vi "nanocal-frontend-server.vi"() -> ()   [LabVIEW 2020]
uses:
  icicle.ctl
  publisher action.ctl
  NanoCalLib 20210521/MCL.lvlibp/SynkTek FPGA/FPGA_SharedResources/FPGASharedResources_Readings_ReadingChannelTypedef.ctl
  NanoCalLib 20210521/MCL.lvlibp/SynkTek FPGA/FPGA_SharedResources/FPGASharedResources_Lockin_Typedef.ctl
  NanoCalLib 20210521/MCL.lvlibp/SynkTek FPGA/FPGA_SharedResources/FPGASharedResources_PhaseType_Typedef.ctl
  NanoCalLib 20210521/NanoCalLib.lvlibp
  NanoCalLib 20210521/MCL.lvlibp/SynkTek FPGA/FPGA_SharedResources/FPGA_SharedResources.lvlib
  NanoCalLib 20210521/MCL.lvlibp
panel:
  in  "Tab Control":enum32{"Page 1", "Page 2"}(tab)
  in  "wait (ms)":u32=50
  out "nanocal data":T1[](array[typedef])=[{"name"="frequency", "units"="Hz", "data"=22.999983439900642}, {"name"="Cs/T", "units"="J/K^2", "data"=3.7739249893269324e-24}, {"name"="Ts", "units"="K", "data"=0.01038672245174747}, {"name"="Ts^2", "units"="K^2", "data"=0.00010788400328963498}, {"name"="Tr", "units"="K", "data"=0.010160855980464388}, {"name"="Cs", "units"="J/K", "data"=3.9198711417852884e-26}, {"name"="Cr", "units"="J/K", "data"=-2.0417082109734875e-18}, {"name"="Ks", "units"="W/K", "data"=2.527872170547633e-23}, {"name"="Kr", "units"="W/K", "data"=3.911459306754245e-15}, {"name"="Rs-therm", "units"="Ohm", "data"=81348.62911437088}, {"name"="Rr-therm", "units"="Ohm", "data"=196009.13306498667}, {"name"="Cr/T", "units"="J/K^2", "data"=-2.0093860348960226e-16}, {"name"="dlogR/dlogT -- S ", "units"="a.u.", "data"=0.8738049990739949}, {"name"="tau", "units"="s", "data"=0.001550660348832471}, {"name"="tan(phi)", "units"="a.u", "data"=0.4481816480367121}, {"name"="Ts,ac", "units"="K", "data"=0.1660718459124116}, {"name"="Tr,ac", "units"="K", "data"=0.0}, {"name"="Hs,ac,out", "units"="V", "data"=0.0}, {"name"="Offset,dc,out", "units"="V", "data"=1.0000000009313226}, {"name"="Vdiff,ac", "units"="V", "data"=4.688238574611993e-09}, {"name"="Vdiff,ac,phase", "units"="deg", "data"=82.61397850464}, {"name"="Stherm,ac,out", "units"="V", "data"=0.0}, {"name"="Rtherm,ac,out", "units"="V", "data"=0.0}, {"name"="CV1 -- Re", "units"="V", "data"=6.026901987025408e-10}, {"name"="CV1 -- Im", "units"="V", "data"=4.649338174070346e-09}, {"name"="DV2 -- Re", "units"="V", "data"=1.0380460195223816e-09}, {"name"="DV2 -- Im", "units"="V", "data"=6.197949303499005e-09}, {"name"="AV2 -- Re", "units"="V", "data"=6.687727898351347e-10}, {"name"="AV2 -- Im", "units"="V", "data"=1.6238645509657183e-10}, {"name"="Vdiff,norm, Re", "units"="V", "data"=1.298136411917629e+18}, {"name"="Vdiff,norm, Im", "units"="V", "data"=1.00142248672243e+19}, {"name"="Resistance.RHr", "units"="ohm", "data"=501162.54690786166}, {"name"="Resistance.RHs", "units"="ohm", "data"=286805.4208747116}]
  in  "Stop":bool
  # "nanocal -- frontend server"
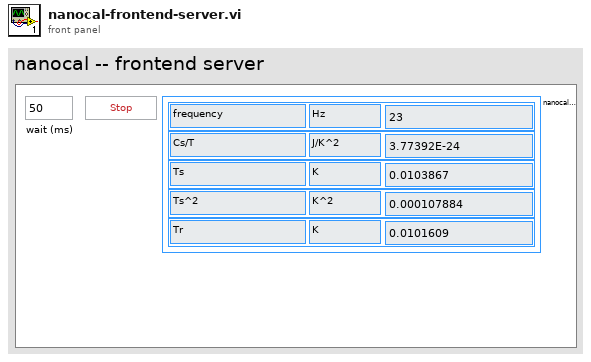
[diagram p1: front panel]
types:
  T1 = typedef "icicle.ctl" = cluster{"name":string, "units":string, "data":dbl}
  T2 = typedef "MCL.lvlibp/MCL_DataRef.ctl" = refnum<vi>
  T3 = typedef "MCL.lvlibp/FPGA_SharedResources.lvlib/FPGASharedResources_PhaseType_Typedef.ctl" = enum16{"DC", "X", "Y", "R", "Theta"}
  T4 = typedef "publisher action.ctl" = enum16{"set", "get", "init", "check"}
  T5 = typedef "MCL.lvlibp/FPGA_SharedResources.lvlib/FPGASharedResources_Lockin_Typedef.ctl" = enum8{"Lock-in set L1", "Lock-in set L2"}
  T6 = typedef "MCL.lvlibp/FPGA_SharedResources.lvlib/FPGASharedResources_Readings_ReadingChannelTypedef.ctl" = enum8{"A V1", "A V2", "B V1", "B V2", "C V1", "C V2", "D V1", "D V2", "E V1", "E V2", "A I", "B I", "C I", "D I", "E I", "Int."}
  T7 = typedef "NanoCalLib.lvlibp/NanoReadings.lvlib/NanoReadings_Parameters_TypeDef.ctl" = cluster{"Power":T8, "C and K":T9, "IV dc":T10, "Tdc,Tac":T11, "Phases":T12, "f etc":T13, "IV 1st harm":T14, "ForAveraging":cluster{"SinTherm":dbl[], "CosTherm":dbl[], "SinHeats":dbl[], "CosHeats":dbl[]}, "Output":T15, "Magnetic field etc.":T16, "Calibration":T17, "CT etc":T18, "IV 2nd harm":T19, "Resistance":T20, "Time etc":T21}
  T8 = typedef "NanoCalLib.lvlibp/NanoReadings.lvlib/NanoReadings_Power.ctl" = cluster{"PHs (W)":dbl, "PHr (W)":dbl, "Ps,dc (W)":dbl, "Pr,dc (W)":dbl, "PHs,dc (W)":dbl, "PHr,dc (W)":dbl, "Ps,ac (W)":dbl, "Pr,ac (W)":dbl, "PHs/PHr":dbl, "Poffs (W)":dbl, "Ps total (W)":dbl, "Pr total (W)":dbl, "Ps-Pr total (W)":dbl, "Ps,offs (W)":dbl, "Ps,cond (W)":dbl, "Ps,net (W)":dbl}
  T9 = typedef "NanoCalLib.lvlibp/NanoReadings.lvlib/NanoReadings_CandK.ctl" = cluster{"Cs (J/K)":dbl, "Ks (W/K)":dbl, "Cr (J/K)":dbl, "Kr (W/K)":dbl, "Cdiff (J/K)":dbl, "Cs-Cr (J/K)":dbl, "Cdiff old style (J/K)":dbl, "Cr from S,diff (J/K)":dbl, "Cs from dT/dt (J/K)":dbl, "Ks,nom (W/K)":dbl}
  T10 = typedef "NanoCalLib.lvlibp/NanoReadings.lvlib/NanoReadings_IandV.ctl" = cluster{"Is,dc (A)":dbl, "Ir,dc (A)":dbl, "Us,dc (V)":dbl, "Ur,dc (V)":dbl, "Udiff,dc (V)":dbl, "IHs dc (A)":dbl, "UHs dc (V)":dbl, "IHr dc (A)":dbl, "UHr dc (V)":dbl, "Uoffs dc (V)":dbl, "Ioffs dc (A)":dbl}
  T11 = typedef "NanoCalLib.lvlibp/NanoReadings.lvlib/NanoReadings_TdcTac.ctl" = cluster{"Ts (K)":dbl, "Tr (K)":dbl, "Tdiff from Rs,Rr":dbl, "Tdiff from Udiff (K)":dbl, "Ts,ac (K)":dbl, "Tr,ac (K)":dbl, "Tdiff,ac (K)":dbl, "Ts,ac driftcorr (K)":dbl, "Tr,ac driftcorr (K)":dbl, "Tr,ac from Ts,diff,ac (K)":dbl, "T target (K)":dbl, "Ts^2 (K^2)":dbl, "Tr^2 (K^2)":dbl, "Tcos/(P/K)":dbl, "Tsin/(P/K)":dbl}
  T12 = typedef "NanoCalLib.lvlibp/NanoReadings.lvlib/NanoReadings_Phases.ctl" = cluster{"Phi Is (deg)":dbl, "Phi Us (deg)":dbl, "Phi Ir (deg)":dbl, "Phi Ur (deg)":dbl, "Phi Udiff (deg)":dbl, "Phi IHs (deg)":dbl, "Phi UHs (deg)":dbl, "Phi IHr (deg)":dbl, "Phi UHr (deg)":dbl, "Phi R from S,diff (deg)":dbl, "Phi Is 1st (deg)":dbl, "Phi Us 1st (deg)":dbl, "Phi Ir 1st (deg)":dbl, "Phi Ur 1st (deg)":dbl, "Phi Udiff 1st (deg)":dbl, "Phi Udiff, raw (deg)":dbl, "S phase (deg)":dbl, "R phase (deg)":dbl, "Diff phase (deg)":dbl}
  T13 = typedef "NanoCalLib.lvlibp/NanoReadings.lvlib/NanoReadings_Frequencies.ctl" = cluster{"f (Hz)":dbl, "f therm (Hz)":dbl, "omega (rad/s)":dbl, "Tan Phi S/diff":dbl, "Sin Phi":dbl, "Cos Phi":dbl, "f mix (Hz)":dbl, "tau (s)":dbl}
  T14 = typedef "NanoCalLib.lvlibp/NanoReadings.lvlib/NanoReadings_FirstHarmonic.ctl" = cluster{"Is,ac 1st (A)":dbl, "Ir,ac 1st (A)":dbl, "Us,ac 1st (V)":dbl, "Ur,ac 1st (V)":dbl, "Udiff,ac 1st (V)":dbl, "IHs (A)":dbl, "UHs (V)":dbl, "IHr (A)":dbl, "UHr (V)":dbl}
  T15 = typedef "NanoCalLib.lvlibp/NanoReadings.lvlib/NanoReadings_Output.ctl" = cluster{"S out phase (deg)":dbl, "R out phase (deg)":dbl, "Hs ac out (Vrms)":dbl, "Hr ac out (Vrms)":dbl, "S Therm dc out (V)":dbl, "R Therm dc out (V)":dbl, "S Therm ac out (Vrms)":dbl, "R Therm ac out (Vrms)":dbl, "Offset dc out (V)":dbl, "Hs dc out (V)":dbl, "Hr dc out (V)":dbl, "Offset ac out (Vrms)":dbl}
  T16 = typedef "NanoCalLib.lvlibp/NanoReadings.lvlib/NanoReadings_MagneticFieldEtc.ctl" = cluster{"H (T)":dbl, "T probe (K)":dbl, "Polar angle (deg)":dbl, "Azimuthal angle (deg)":dbl}
  T17 = typedef "NanoCalLib.lvlibp/NanoReadings.lvlib/NanoReadings_Calibration.ctl" = cluster{"1+Rs/RIs factor":dbl, "1+RIs/Rs factor":dbl, "Rs,scaled (ohm)":dbl, "Rr,scaled (ohm)":dbl, "R lead S (ohm)":dbl, "R lead R (ohm)":dbl, "|dlnR/dlnT| S":dbl, "|dlnR/dlnT| R":dbl, "dTs/dt (mK/s)":dbl, "dTr/dt (mK/s)":dbl}
  T18 = typedef "NanoCalLib.lvlibp/NanoReadings.lvlib/NanoReadings_CTetc.ctl" = cluster{"Cs/T (J/K^2)":dbl, "Cr/T (J/K^2)":dbl, "Cdiff/T (J/K^2)":dbl, "(Cs-Cr)/T (J/K^2)":dbl, "Cdiff/T old style (J/K^2)":dbl, "Cr/T from S,diff (J/K^2)":dbl}
  T19 = typedef "NanoCalLib.lvlibp/NanoReadings.lvlib/NanoReadings_2ndHarmonic.ctl" = cluster{"Is,ac (A)":dbl, "Ir,ac (A)":dbl, "Us,ac (V)":dbl, "Ur,ac (V)":dbl, "Udiff,ac (V)":dbl}
  T20 = typedef "NanoCalLib.lvlibp/NanoReadings.lvlib/NanoReadings_Resistance.ctl" = cluster{"RHs (ohm)":dbl, "RHr (ohm)":dbl, "Rs (ohm)":dbl, "Rr (ohm)":dbl, "RHs,dc (ohm)":dbl, "RHr,dc (ohm)":dbl, "Rs,ac (ohm)":dbl, "Rr,ac (ohm)":dbl, "Roffs (ohm)":dbl}
  T21 = typedef "NanoCalLib.lvlibp/NanoReadings.lvlib/NanoReadings_TimeEtc.ctl" = cluster{"Time (s)":dbl, "Datapoint index":dbl, "Datapoint time (s)":dbl}
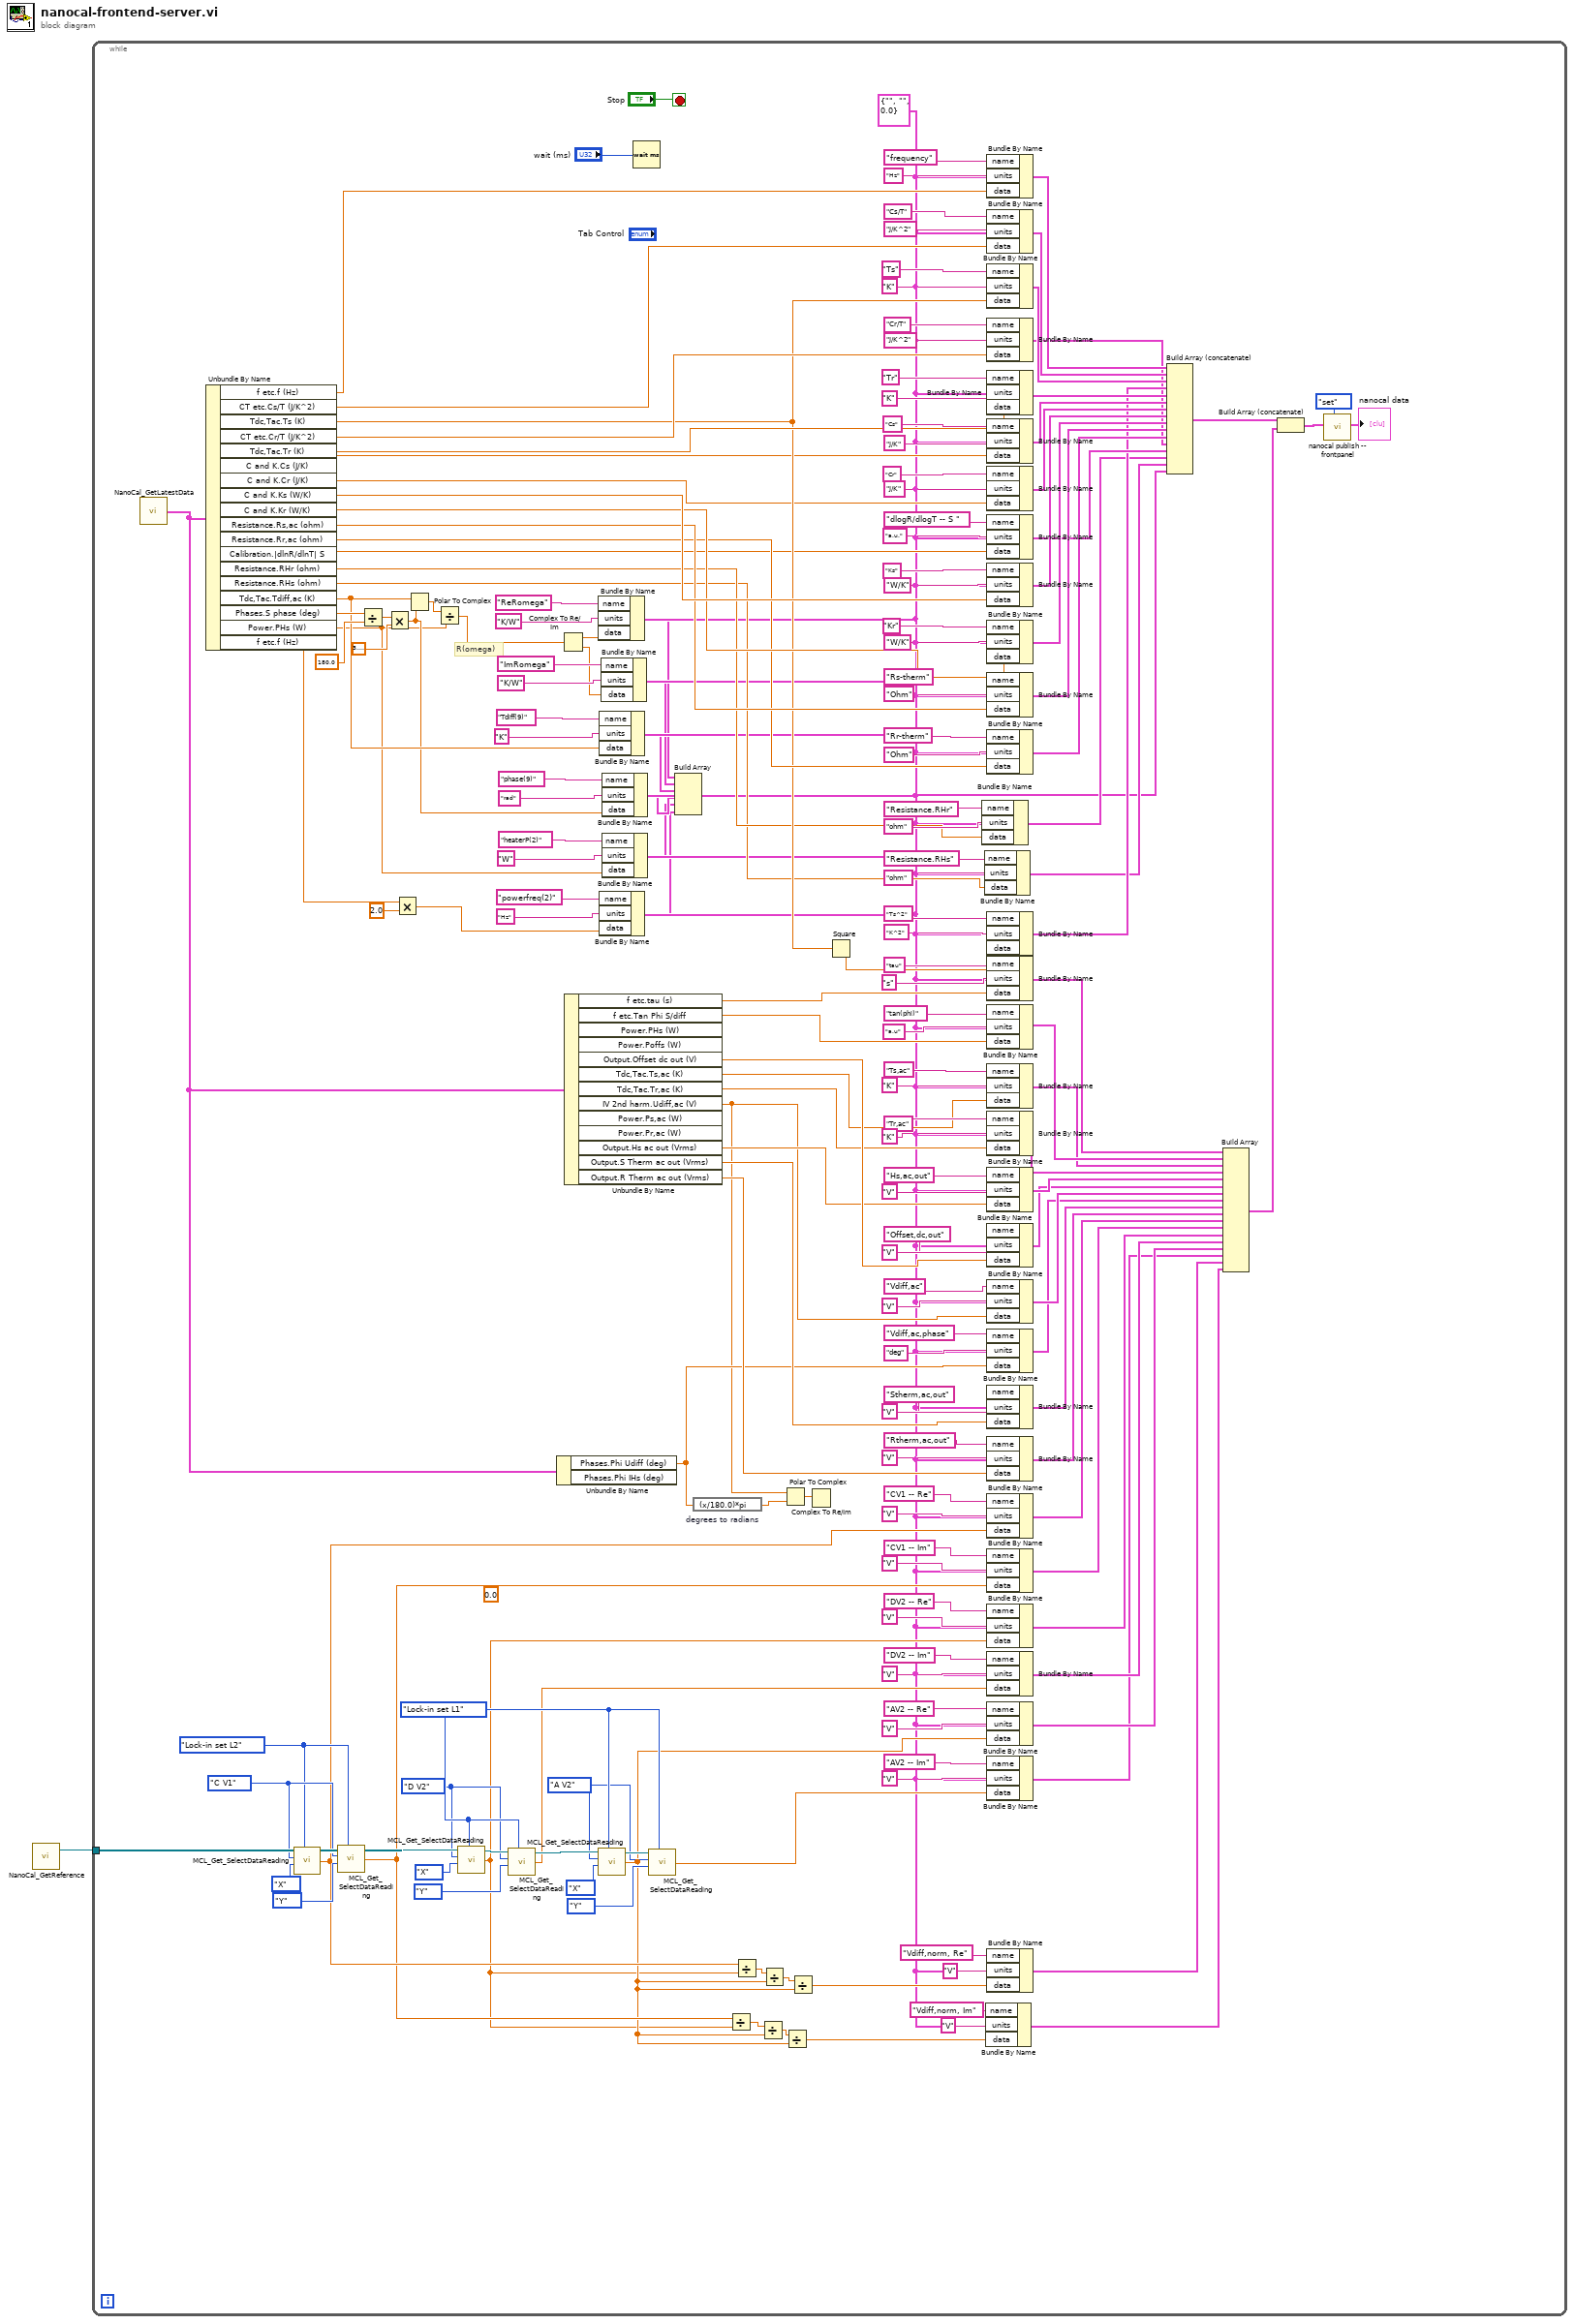
[diagram p0: block diagram]
diagram:
  n1 = call "NanoCal_GetReference.vi"() -> ("Connected MCL object"=w1:T2)  [unwired: 2 in, 1 out]
  n2 = while {
    tunnel: w1 -> [w94]
    stop <- "Stop" stop-if-true
    w85 = FPGASharedResources_Lockin_Typedef."Lock-in set L1" ("Lockin")
    w82 = FPGASharedResources_Readings_ReadingChannelTypedef."A V2" ("Reading Ch")
    w81 = FPGASharedResources_Readings_ReadingChannelTypedef."D V2" ("Reading Ch")
    w92 = FPGASharedResources_Lockin_Typedef."Lock-in set L2" ("Lockin")
    w93 = FPGASharedResources_Readings_ReadingChannelTypedef."C V1" ("Reading Ch")
    (unwired) 0.0 ("Select reading")
    w9 = T1 {"name"="", "units"="", "data"=0.0} ("icicle")
    # "R(omega)"
    n3 = call "NanoCal_GetLatestData.vi"() -> ("Latest data"=w44:T7)  [unwired: 1 in]
    n4 = Unbundle By Name(w44) -> ("f etc.f (Hz)"=w193:dbl, "CT etc.Cs/T (J/K^2)"=w185:dbl, "Tdc,Tac.Ts (K)"=w157:dbl, "CT etc.Cr/T (J/K^2)"=w186:dbl, "Tdc,Tac.Tr (K)"=w180:dbl, "C and K.Cs (J/K)"=w151:dbl, "C and K.Cr (J/K)"=w150:dbl, "C and K.Ks (W/K)"=w176:dbl, "C and K.Kr (W/K)"=w170:dbl, "Resistance.Rs,ac (ohm)"=w162:dbl, "Resistance.Rr,ac (ohm)"=w161:dbl, "Calibration.|dlnR/dlnT| S"=w48:dbl, "Resistance.RHr (ohm)"=w39:dbl, "Resistance.RHs (ohm)"=w38:dbl, "Tdc,Tac.Tdiff,ac (K)"=w19:dbl, "Phases.S phase (deg)"=w34:dbl, "Power.PHs (W)"=w15:dbl, "f etc.f (Hz)"=w12:dbl)
    n5 = call "MCL_Get_SelectDataReading.vi"("MCL object"=w94, "Reading Ch"=w93, "PhaseType"=FPGASharedResources_PhaseType_Typedef."X", "Lockin"=w92) -> ("MCL object"=w95:T2, "Select reading"=w62:dbl)  [unwired: 1 in, 1 out]
    n6 = call "MCL_Get_SelectDataReading.vi"("MCL object"=w95, "Reading Ch"=w93, "PhaseType"=FPGASharedResources_PhaseType_Typedef."Y", "Lockin"=w92) -> ("MCL object"=w89:T2, "Select reading"=w56:dbl)  [unwired: 1 in, 1 out]
    n7 = Divide(x=w34, y=180.0) -> (x/y=w35:dbl)
    n8 = Multiply(x=w35, y=3.141592653589793) -> (x*y=w18:dbl)
    n9 = Multiply(x=w12, y=2.0) -> (x*y=w10:dbl)
    n10 = Polar To Complex(1:w18, 2:w19) -> (0:w31:cdb)
    n11 = Divide(x=w31, y=w15) -> (x/y=w26:cdb)
    n12 = call "MCL_Get_SelectDataReading.vi"("MCL object"=w89, "Reading Ch"=w81, "PhaseType"=FPGASharedResources_PhaseType_Typedef."X", "Lockin"=w85) -> ("MCL object"=w88:T2, "Select reading"=w53:dbl)  [unwired: 1 in, 1 out]
    n13 = call "MCL_Get_SelectDataReading.vi"("MCL object"=w88, "Reading Ch"=w81, "PhaseType"=FPGASharedResources_PhaseType_Typedef."Y", "Lockin"=w85) -> ("MCL object"=w87:T2, "Select reading"=w67:dbl)  [unwired: 1 in, 1 out]
    n14 = Unbundle By Name(w44) -> ("Phases.Phi Udiff (deg)"=w107:dbl)  [unwired: 1 out]
    n15 = Complex To Re/Im(x + iy=w26) -> (x=w25:dbl, y=w24:dbl)
    n16 = Unbundle By Name(w44) -> ("f etc.tau (s)"=w140:dbl, "f etc.Tan Phi S/diff"=w132:dbl, "Output.Offset dc out (V)"=w137:dbl, "Tdc,Tac.Ts,ac (K)"=w136:dbl, "Tdc,Tac.Tr,ac (K)"=w135:dbl, "IV 2nd harm.Udiff,ac (V)"=w105:dbl, "Output.Hs ac out (Vrms)"=w131:dbl, "Output.S Therm ac out (Vrms)"=w116:dbl, "Output.R Therm ac out (Vrms)"=w115:dbl)  [unwired: 4 out]
    n17 = Bundle By Name(cluster=w9, "name"="ReRomega", "units"="K/W", "data"=w25) -> (w7:T1)
    n18 = call "MCL_Get_SelectDataReading.vi"("MCL object"=w87, "Reading Ch"=w82, "PhaseType"=FPGASharedResources_PhaseType_Typedef."X", "Lockin"=w85) -> ("MCL object"=w86:T2, "Select reading"=w54:dbl)  [unwired: 1 in, 1 out]
    n19 = Bundle By Name(cluster=w9, "name"="Tdiff(9)", "units"="K", "data"=w19) -> (w6:T1)
    n20 = Bundle By Name(cluster=w9, "name"="powerfreq(2)", "units"="Hz", "data"=w10) -> (w3:T1)
    n21 = Bundle By Name(cluster=w9, "name"="ImRomega", "units"="K/W", "data"=w24) -> (w8:T1)
    n22 = Bundle By Name(cluster=w9, "name"="phase(9)", "units"="rad", "data"=w18) -> (w5:T1)
    n23 = Bundle By Name(cluster=w9, "name"="heaterP(2)", "units"="W", "data"=w15) -> (w4:T1)
    n24 = Wait (ms)(milliseconds to wait="wait (ms)") -> ()  [unwired: 1 out]
    n25 = call "MCL_Get_SelectDataReading.vi"("MCL object"=w86, "Reading Ch"=w82, "PhaseType"=FPGASharedResources_PhaseType_Typedef."Y", "Lockin"=w85) -> ("Select reading"=w68:dbl)  [unwired: 1 in, 2 out]
    n26 = Build Array(w7, w8, w6, w5, w4, w3) -> (w2:T1[])
    n27 = expression code="(x/180.0)*pi" "degrees to radians"(w107) -> (w108:dbl)
    n28 = Divide(x=w56, y=w53) -> (x/y=w58:dbl)
    n29 = Divide(x=w62, y=w53) -> (x/y=w61:dbl)
    n30 = Divide(x=w58, y=w54) -> (x/y=w57:dbl)
    n31 = Divide(x=w61, y=w54) -> (x/y=w60:dbl)
    n32 = Polar To Complex(1:w108, 2:w105) -> (0:w104:cdb)
    n33 = Divide(x=w57, y=w54) -> (x/y=w55:dbl)
    n34 = Divide(x=w60, y=w54) -> (x/y=w59:dbl)
    n35 = Complex To Re/Im(x + iy=w104) -> ()  [unwired: 2 out]
    n36 = Square(x=w157) -> (x^2=w158:dbl)
    n37 = Bundle By Name(cluster=w9, "name"="Resistance.RHr", "units"="ohm", "data"=w39) -> (w37:T1)
    n38 = Bundle By Name(cluster=w9, "name"="Resistance.RHs", "units"="ohm", "data"=w38) -> (w36:T1)
    n39 = Bundle By Name(cluster=w9, "name"="Vdiff,norm, Im", "units"="V", "data"=w55) -> (w51:T1)
    n40 = Bundle By Name(cluster=w9, "name"="frequency", "units"="Hz", "data"=w193) -> (w182:T1)
    n41 = Bundle By Name(cluster=w9, "name"="Cs/T", "units"="J/K^2", "data"=w185) -> (w183:T1)
    n42 = Bundle By Name(cluster=w9, "name"="Ts", "units"="K", "data"=w157) -> (w184:T1)
    n43 = Bundle By Name(cluster=w9, "name"="Cr/T", "units"="J/K^2", "data"=w186) -> (w45:T1)
    n44 = Bundle By Name(cluster=w9, "name"="Tr", "units"="K", "data"=w180) -> (w179:T1)
    n45 = Bundle By Name(cluster=w9, "name"="Cs", "units"="J/K", "data"=w151) -> (w154:T1)
    n46 = Bundle By Name(cluster=w9, "name"="Cr", "units"="J/K", "data"=w150) -> (w149:T1)
    n47 = Bundle By Name(cluster=w9, "name"="dlogR/dlogT -- S ", "units"="a.u.", "data"=w48) -> (w47:T1)
    n48 = Bundle By Name(cluster=w9, "name"="Ks", "units"="W/K", "data"=w176) -> (w175:T1)
    n49 = Bundle By Name(cluster=w9, "name"="Kr", "units"="W/K", "data"=w170) -> (w169:T1)
    n50 = Bundle By Name(cluster=w9, "name"="Rs-therm", "units"="Ohm", "data"=w162) -> (w164:T1)
    n51 = Bundle By Name(cluster=w9, "name"="Rr-therm", "units"="Ohm", "data"=w161) -> (w163:T1)
    n52 = Bundle By Name(cluster=w9, "name"="Ts^2", "units"="K^2", "data"=w158) -> (w46:T1)
    n53 = Bundle By Name(cluster=w9, "name"="tau", "units"="s", "data"=w140) -> (w130:T1)
    n54 = Bundle By Name(cluster=w9, "name"="tan(phi)", "units"="a.u", "data"=w132) -> (w129:T1)
    n55 = Bundle By Name(cluster=w9, "name"="Ts,ac", "units"="K", "data"=w136) -> (w128:T1)
    n56 = Bundle By Name(cluster=w9, "name"="Tr,ac", "units"="K", "data"=w135) -> (w127:T1)
    n57 = Bundle By Name(cluster=w9, "name"="Hs,ac,out", "units"="V", "data"=w131) -> (w126:T1)
    n58 = Bundle By Name(cluster=w9, "name"="Offset,dc,out", "units"="V", "data"=w137) -> (w125:T1)
    n59 = Bundle By Name(cluster=w9, "name"="Vdiff,ac", "units"="V", "data"=w105) -> (w114:T1)
    n60 = Bundle By Name(cluster=w9, "name"="Vdiff,ac,phase", "units"="deg", "data"=w107) -> (w111:T1)
    n61 = Bundle By Name(cluster=w9, "name"="Stherm,ac,out", "units"="V", "data"=w116) -> (w112:T1)
    n62 = Bundle By Name(cluster=w9, "name"="Rtherm,ac,out", "units"="V", "data"=w115) -> (w113:T1)
    n63 = Bundle By Name(cluster=w9, "name"="CV1 -- Re", "units"="V", "data"=w62) -> (w99:T1)
    n64 = Bundle By Name(cluster=w9, "name"="CV1 -- Im", "units"="V", "data"=w56) -> (w98:T1)
    n65 = Bundle By Name(cluster=w9, "name"="DV2 -- Re", "units"="V", "data"=w53) -> (w72:T1)
    n66 = Bundle By Name(cluster=w9, "name"="DV2 -- Im", "units"="V", "data"=w67) -> (w71:T1)
    n67 = Bundle By Name(cluster=w9, "name"="AV2 -- Re", "units"="V", "data"=w54) -> (w70:T1)
    n68 = Bundle By Name(cluster=w9, "name"="AV2 -- Im", "units"="V", "data"=w68) -> (w69:T1)
    n69 = Bundle By Name(cluster=w9, "name"="Vdiff,norm, Re", "units"="V", "data"=w59) -> (w52:T1)
    n70 = Build Array (concatenate)(w182, w183, w184, w46, w179, w154, w149, w175, w169, w164, w163, w45, w47, w37, w36, w2) -> (w124:T1[])
    n71 = Build Array(w130, w129, w128, w127, w126, w125, w114, w111, w112, w113, w99, w98, w72, w71, w70, w69, w52, w51) -> (w123:T1[])
    n72 = Build Array (concatenate)(w124, w123) -> (w122:T1[])
    n73 = call "nanocal publish -- frontpanel.vi"("publisher action"=publisher_action."set", "nanocal data array IN"=w122) -> ("nanocal data array OUT"=→"nanocal data":T1[])  [unwired: 9 in]
  }
